vi "calc.vi"() -> ()   [LabVIEW 2011]
uses:
  global_vars.vi
  <vilib>/Utility/file.llb/Write To Spreadsheet File (I64).vi
panel:
  in  "b_calc_all":bool
  out "calculating":bool
  in  "calc \ndisplacement":bool
  in  "file path (dialog if empty)":path
  in  "dbl_gamma_correction":dbl=1.0
  in  "dbl_noise_threshold":dbl=20.0
  in  "update global variables":bool
  in  "safety margin":i32=5
  out "u8_ar_noise_mask":u8[][](array[numeric])
  in  "Tab Control":T1(tab)
  out "img_dist_input":T2(plugin-control)
  out "img_orig_input":T2(plugin-control)
  in  "i32_sel_input_image":i32
  in  "select row input":i32(slide) scale=-1.1..1049.0
  out "input_line_plot":dbl[][](graph)
  out "noise_mask_line_plot":u8[](graph)
  in  "select row noise map":i32(slide) scale=-1.1..1049.0
  out "last px":i32
  out "first px":i32
  out "img_noise_mask":T2(plugin-control)
  out "i32_First/last px":i32[][](graph)
  out "lineplot phasemap":dbl[][](graph)
  in  "select row phasemap":i32(slide) scale=0.0..1049.0
  out "img_dist_phaseMap":T2(plugin-control)
  out "img_orig_masked_with_dist":T2(plugin-control)
  out "img_dist_unwrap":T2(plugin-control)
  out "img_orig_unwrap":T2(plugin-control)
  in  "select row unwrapped":i32(slide) scale=-1.1..1049.0
  out "lineplot unwrapped":dbl[][](graph)
  out "graph_displacement":i32[][](graph)
  in  "select row displacement":i32(slide) scale=-1.1..1049.0
  out "lineplot displacement":i32[](graph)
  in  "save data":bool
  out "i32_ar_displacement":i32[][](array[numeric])
  in  "calc \nunwrapped\nphase map":bool
  out "Y Resolution":i32
  out "X Resolution":i32
  in  "update_cor":bool
  out "path_dist_files":path[](array[path])=[path "X:/Cloud Drives/Dropbox/Europhotonics/FringeMan/Image Storage/02_07/x-direction/dist/12_56_10-5.00fringes_0of4__capt_.png", path "X:/Cloud Drives/Dropbox/Europhotonics/FringeMan/Image Storage/02_07/x-direction/dist/12_56_10-5.00fringes_1of4__capt_.png", path "X:/Cloud Drives/Dropbox/Europhotonics/FringeMan/Image Storage/02_07/x-direction/dist/12_56_10-5.00fringes_2of4__capt_.png", path "X:/Cloud Drives/Dropbox/Europhotonics/FringeMan/Image Storage/02_07/x-direction/dist/12_56_10-5.00fringes_3of4__capt_.png"]
  out "path_orig_files":path[](array[path])=[path "X:/Cloud Drives/Dropbox/Europhotonics/FringeMan/Image Storage/02_07/x-direction/orig/12_56_10-5.00fringes_0of4__original_.png", path "X:/Cloud Drives/Dropbox/Europhotonics/FringeMan/Image Storage/02_07/x-direction/orig/12_56_10-5.00fringes_1of4__original_.png", path "X:/Cloud Drives/Dropbox/Europhotonics/FringeMan/Image Storage/02_07/x-direction/orig/12_56_10-5.00fringes_2of4__original_.png", path "X:/Cloud Drives/Dropbox/Europhotonics/FringeMan/Image Storage/02_07/x-direction/orig/12_56_10-5.00fringes_3of4__original_.png"]
  in  "dbl_ar_crop_correction":dbl[](array[numeric])=[0.0, 0.0, 0.0, 0.0] caption="crop_correction"
  in  "u8_y_center_cor":i16
  in  "u8_x_center_cor":i16=-20
  in  "radius correction":i16=-30
  out "u8_ar_orig_phasemap":dbl[][](array[numeric])
  out "dbl_pxar_orig_unwrap":dbl[][](array[numeric])
  out "dbl_pxar_dist_unwrap":dbl[][](array[numeric])
  out "u8_pxar_orig":dbl[][][](array[numeric])
  in  "read orig":bool
  in  "read dist":bool
  out "u8_ar_dist_phasemap":dbl[][](array[numeric])
  in  "calculate \nphase map":bool
  out "u8_pxar_dist":dbl[][][](array[numeric])
  in  "Stop Button":bool
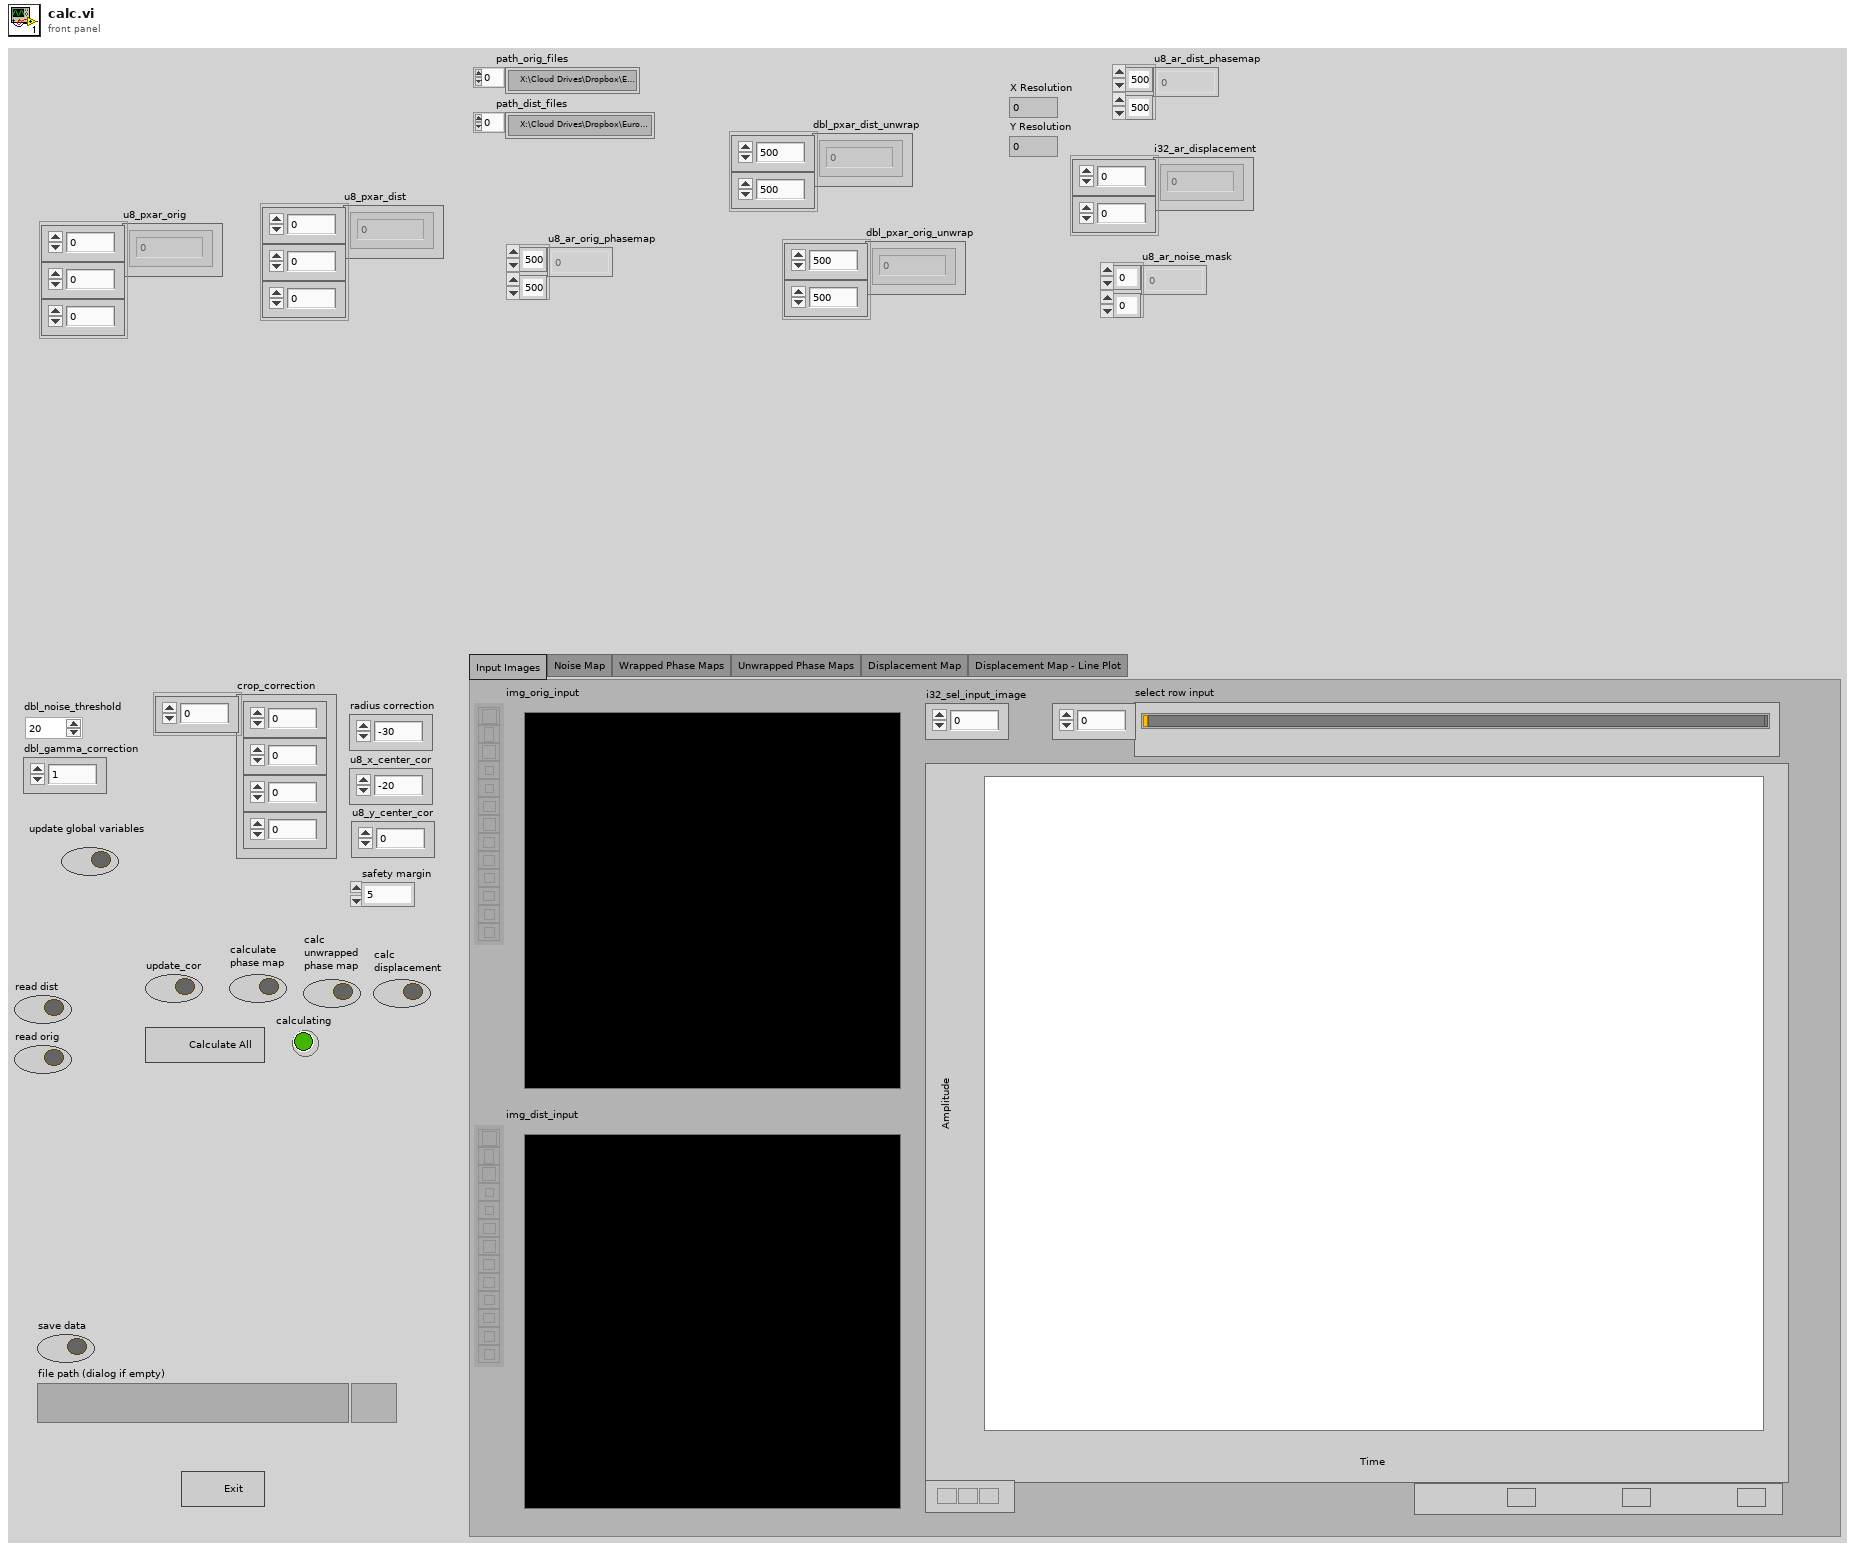
[diagram p1: front panel]
types:
  T1 = enum32{"Input Images", "Noise Map", "Wrapped Phase Maps", "Unwrapped Phase Maps", "Displacement Map", "Displacement Map - Line Plot"}
  T2 = typedef "IMAQ Image.ctl" = refnum<image>
  T3 = cluster{"radius correction":i16, "u8_x_center_cor":i16, "u8_y_center_cor":i16}
  T4 = typedef "Image Type" = u32
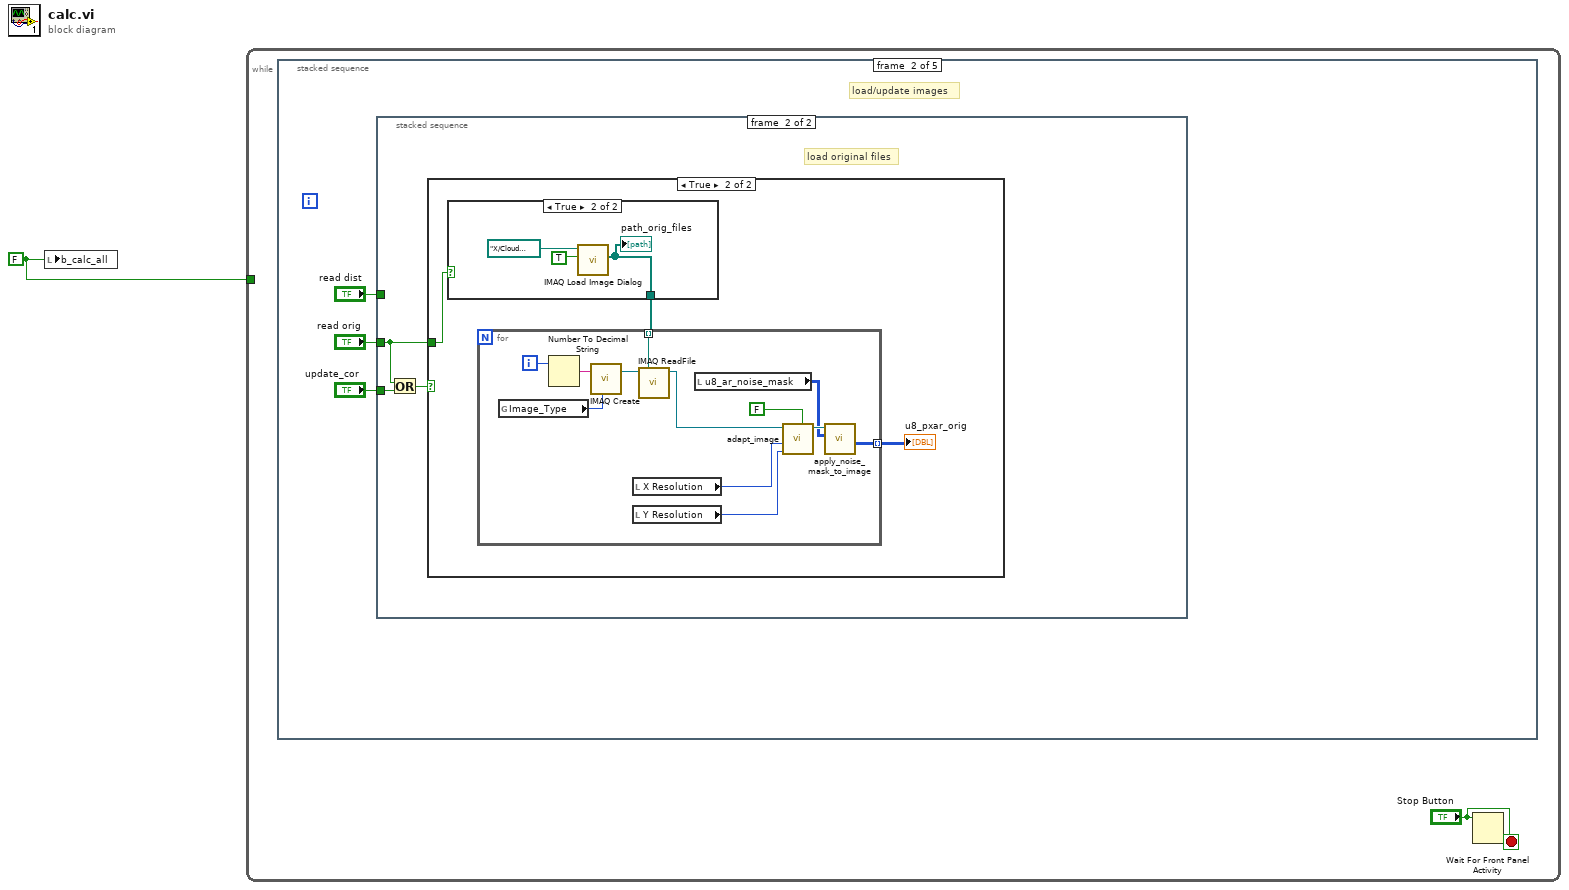
[diagram p0: block diagram]
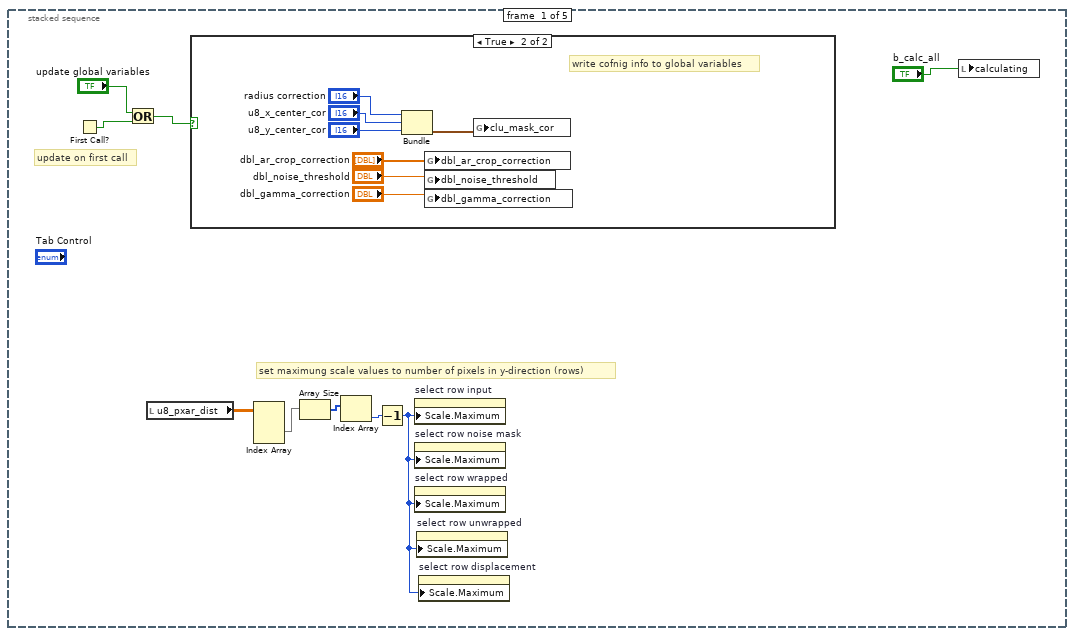
[diagram p2: hidden frame]
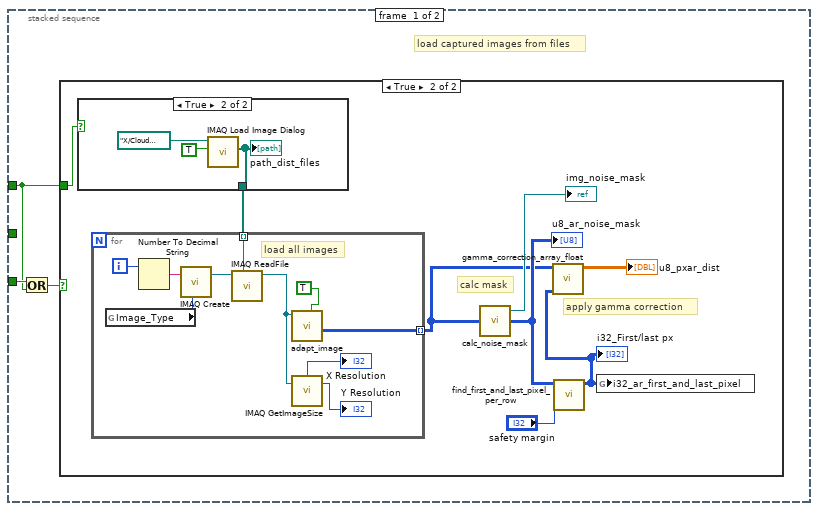
[diagram p4: hidden frame]
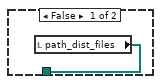
[diagram p6: hidden frame]
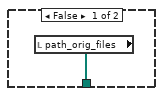
[diagram p8: hidden frame]
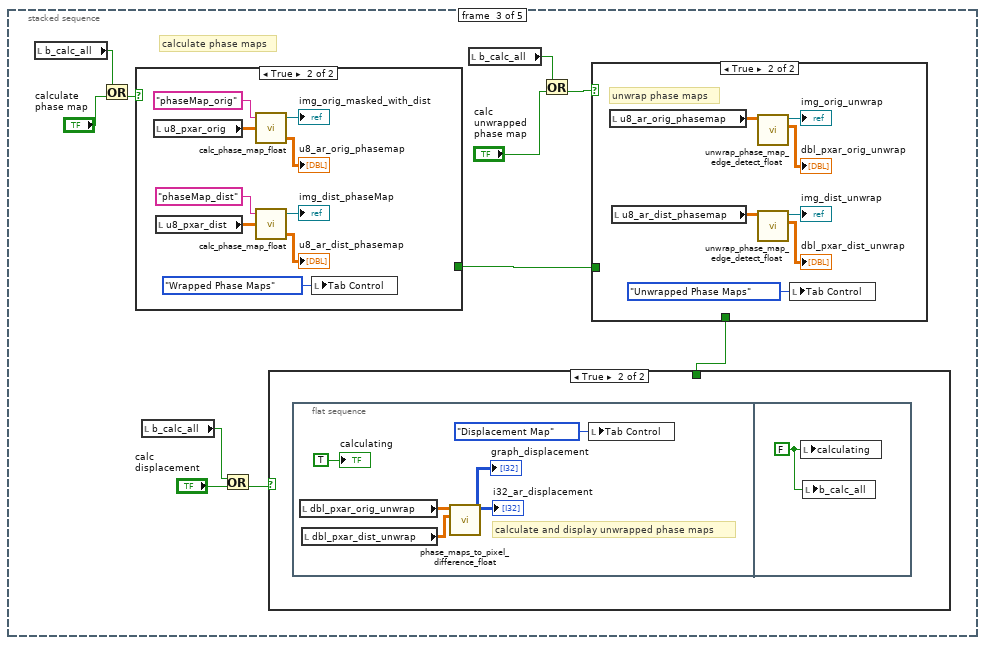
[diagram p9: hidden frame]
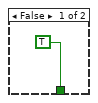
[diagram p11: hidden frame]
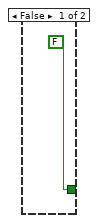
[diagram p12: hidden frame]
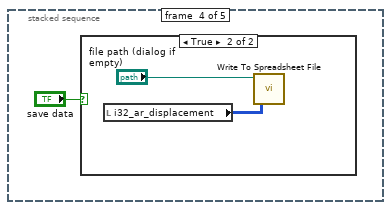
[diagram p13: hidden frame]
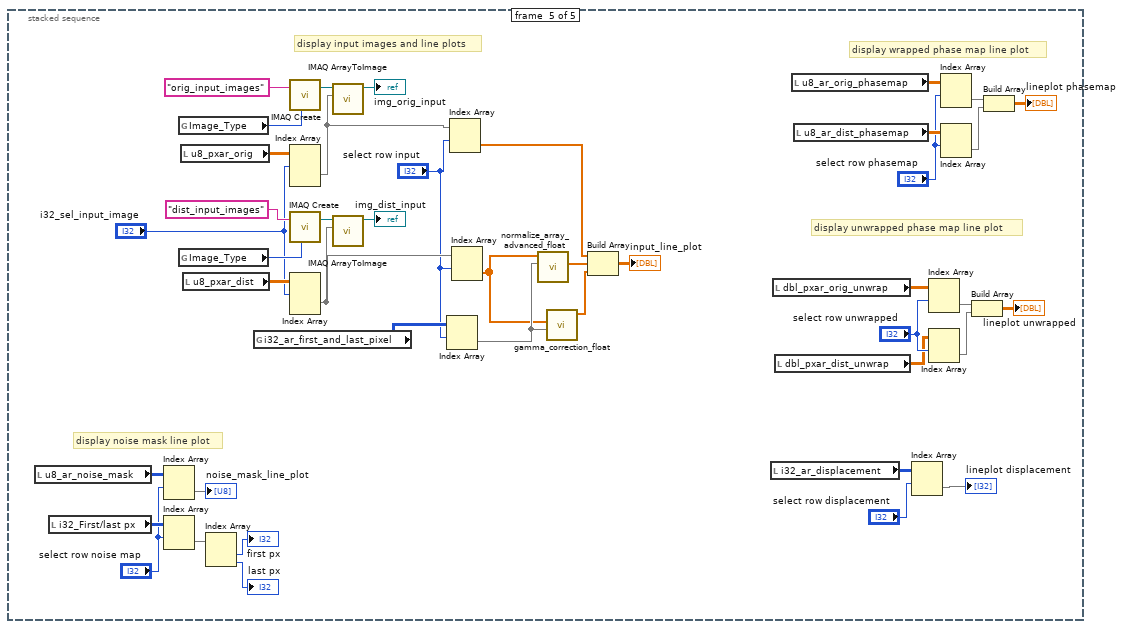
[diagram p15: hidden frame]
diagram:
  w1 = FALSE ("b_calculate all")
  n1 = local write "b_calc_all"(w1) -> ()
  n2 = while {
    tunnel: w1 -> [_]
    stop <- "Stop Button" stop-if-true
    n3 = stacked-sequence {
      frame #0 {
        # "set maximung scale values to number of pixels in y-direction (rows)"
        # "update on first call"
        n4 = First Call?() -> (First Call?: T/F=w9:bool)
        n5 = Or(x="update global variables", y=w9) -> (x .or. y?=w10:bool)
        n6 = local read "u8_pxar_dist"() -> (w7:dbl[][][])
        n7 = case shown="True" w10 {
          frame False {
          }
          frame True {
            # "write cofnig info to global variables"
            n8 = Bundle("radius correction"="radius correction", "u8_x_center_cor"="u8_x_center_cor", "u8_y_center_cor"="u8_y_center_cor") -> (w18:T3)  [unwired: 1 in]
            n9 = global write "global_vars.vi" "dbl_ar_crop_correction"("dbl_ar_crop_correction") -> ()
            n10 = global write "global_vars.vi" "dbl_noise_threshold"("dbl_noise_threshold") -> ()
            n11 = global write "global_vars.vi" "dbl_gamma_correction"("dbl_gamma_correction") -> ()
            n12 = global write "global_vars.vi" "clu_mask_cor"(w18) -> ()
          }
        }
        n13 = Index Array(array=w7) -> (element=w8:dbl[][])  [unwired: 3 in]
        n14 = Array Size(array=w8) -> (size(s)=w6:i32[])
        n15 = Index Array(array=w6) -> (element=w5:i32)  [unwired: 1 in]
        n16 = Decrement(x=w5) -> (x-1=w4:i32)
        n17 = property on="select row input" class="Slide (strict)"("Scale.Maximum"=w4) -> ()  [unwired: 2 in, 2 out]
        n18 = property on="select row noise mask" class="Slide (strict)"("Scale.Maximum"=w4) -> ()  [unwired: 2 in, 2 out]
        n19 = property on="select row wrapped" class="Slide (strict)"("Scale.Maximum"=w4) -> ()  [unwired: 2 in, 2 out]
        n20 = property on="select row unwrapped" class="Slide (strict)"("Scale.Maximum"=w4) -> ()  [unwired: 2 in, 2 out]
        n21 = property on="select row displacement" class="Slide (strict)"("Scale.Maximum"=w4) -> ()  [unwired: 2 in, 2 out]
        n22 = local write "calculating"("b_calc_all") -> ()
      }
      frame #1 {
        # "load/update images"
        n23 = stacked-sequence {
          tunnel: "update_cor" -> [w24 w48]
          tunnel: "read dist" -> [w22 _]
          tunnel: "read orig" -> [_ w47]
          frame #0 {
            # "load captured images from files"
            n24 = Or(x=w24, y=w22) -> (x .or. y?=w23:bool)
            n25 = case shown="True" w23 {
              tunnel: w22 -> [_ w31]
              frame False {
              }
              frame True {
                # "apply gamma correction"
                # "calc mask"
                n26 = case shown="True" w31 {
                  tunnel: [w33 w36] -> w32
                  frame False {
                    n27 = local read "path_dist_files"() -> (w33:path[])
                  }
                  frame True {
                    n28 = call "IMAQ Load Image Dialog"("Multiple Files? (No)"=TRUE, "Start Path"=path "X:/Cloud Drives/Dropbox/Europhotonics/FringeMan/Image Storage") -> ("Paths"=w36:path[])  [unwired: 7 in, 2 out]
                    "path_dist_files" <- w36
                  }
                }
                n29 = for {
                  tunnel: w32 -> [w42] mode=indexing
                  tunnel: [w38] -> w27 mode=indexing
                  i -> [w46]
                  # "load all images"
                  n30 = global read "global_vars.vi" "Image_Type"() -> (w43:T4)
                  n31 = Number To Decimal String(number=w46) -> (decimal integer string=w45:string)  [unwired: 1 in]
                  n32 = call "IMAQ Create"("Image Name"=w45, "Image Type"=w43) -> ("New Image"=w44:T2)  [unwired: 2 in, 2 out]
                  n33 = call "IMAQ ReadFile"("File Path"=w42, "Image"=w44) -> ("Image Out"=w39:T2)  [unwired: 5 in, 4 out]
                  n34 = call "adapt_image.vi"("captured image?"=TRUE, "orig_imageIn"=w39) -> ("adapted image px array"=w38:u8[][])  [unwired: 7 in, 2 out]
                  n35 = call "IMAQ GetImageSize"("Image"=w39) -> ("Y Resolution"=→"Y Resolution":i32, "X Resolution"=→"X Resolution":i32)  [unwired: 3 in, 1 out]
                }
                n36 = call "calc_noise_mask.vi"("u8_ar_image_pixel_array"=w27) -> ("u8_ar_noise_mask"=w28:u8[][], "img_noise mask"=→"img_noise_mask":T2)  [unwired: 3 in]
                "u8_ar_noise_mask" <- w28
                n37 = call "find_first_and_last_pixel_per_row.vi"("safety margin"="safety margin", "u8_ar_mask"=w28) -> ("i32_ar_first_and_last_pixel"=w25:i32[][])  [unwired: 9 in]
                "i32_First/last px" <- w25
                n38 = call "gamma_correction_array_float.vi"("i32_ar_first_and_last_pixel"=w25, "adapted image px array"=w27) -> ("i16_normalized unwrapped array"=→"u8_pxar_dist":dbl[][][])  [unwired: 9 in]
                n39 = global write "global_vars.vi" "i32_ar_first_and_last_pixel"(w25) -> ()
              }
            }
          }
          frame #1 {
            # "load original files"
            n40 = Or(x=w47, y=w48) -> (x .or. y?=w49:bool)
            n41 = case shown="True" w49 {
              tunnel: w47 -> [_ w51]
              frame False {
              }
              frame True {
                n42 = case shown="True" w51 {
                  tunnel: [w53 w55] -> w52
                  frame False {
                    n43 = local read "path_orig_files"() -> (w53:path[])
                  }
                  frame True {
                    n44 = call "IMAQ Load Image Dialog"("Multiple Files? (No)"=TRUE, "Start Path"=path "X:/Cloud Drives/Dropbox/Europhotonics/FringeMan/Image Storage") -> ("Paths"=w55:path[])  [unwired: 7 in, 2 out]
                    "path_orig_files" <- w55
                  }
                }
                n45 = for {
                  tunnel: w52 -> [w68] mode=indexing
                  tunnel: [w58] -> w50 mode=indexing
                  i -> [w64]
                  n46 = global read "global_vars.vi" "Image_Type"() -> (w65:T4)
                  n47 = Number To Decimal String(number=w64) -> (decimal integer string=w67:string)  [unwired: 1 in]
                  n48 = call "IMAQ Create"("Image Name"=w67, "Image Type"=w65) -> ("New Image"=w66:T2)  [unwired: 2 in, 2 out]
                  n49 = local read "X Resolution"() -> (w62:i32)
                  n50 = local read "Y Resolution"() -> (w61:i32)
                  n51 = call "IMAQ ReadFile"("File Path"=w68, "Image"=w66) -> ("Image Out"=w63:T2)  [unwired: 5 in, 4 out]
                  n52 = local read "u8_ar_noise_mask"() -> (w57:u8[][])
                  n53 = call "adapt_image.vi"("captured image?"=FALSE, "captImage_Y_Resolution"=w61, "captImage_X_Resolution"=w62, "orig_imageIn"=w63) -> ("adapted image"=w59:T2)  [unwired: 5 in, 2 out]
                  n54 = call "apply_noise_mask_to_image.vi"("u8_ar_noise_mask in"=w57, "Refnum in"=w59) -> ("Image Pixels (U8)"=w58:u8[][])  [unwired: 7 in, 2 out]
                }
                "u8_pxar_orig" <- w50
              }
            }
          }
        }
      }
      frame #2 {
        # "calculate phase maps"
        n55 = local read "b_calc_all"() -> (w71:bool)
        n56 = Or(x=w71, y="calculate \nphase map") -> (x .or. y?=w74:bool)
        n57 = case shown="True" w74 {
          tunnel: [FALSE _] -> w77
          frame False {
          }
          frame True {
            n58 = local read "u8_pxar_orig"() -> (w98:dbl[][][])
            n59 = local read "u8_pxar_dist"() -> (w102:dbl[][][])
            n60 = call "calc_phase_map_float.vi"("u8_ar_image_pixel_array"=w98, "image name"="phaseMap_orig" ("String")) -> ("raw phase map array"=→"u8_ar_orig_phasemap":dbl[][], "phase map"=→"img_orig_masked_with_dist":T2)  [unwired: 2 in]
            n61 = call "calc_phase_map_float.vi"("u8_ar_image_pixel_array"=w102, "image name"="phaseMap_dist" ("String")) -> ("raw phase map array"=→"u8_ar_dist_phasemap":dbl[][], "phase map"=→"img_dist_phaseMap":T2)  [unwired: 2 in]
            n62 = local write "Tab Control"(T1."Wrapped Phase Maps" ("Tab Control")) -> ()
          }
        }
        n63 = local read "b_calc_all"() -> (w69:bool)
        n64 = Or(x=w69, y="calc \ndisplacement") -> (x .or. y?=w72:bool)
        n65 = local read "b_calc_all"() -> (w70:bool)
        n66 = Or(x=w70, y="calc \nunwrapped\nphase map") -> (x .or. y?=w73:bool)
        n67 = case shown="True" w73 {
          tunnel: w77 -> [_ _]
          tunnel: [TRUE _] -> w75
          frame False {
          }
          frame True {
            # "unwrap phase maps"
            n68 = local read "u8_ar_orig_phasemap"() -> (w90:dbl[][])
            n69 = local read "u8_ar_dist_phasemap"() -> (w91:dbl[][])
            n70 = call "unwrap_phase_map_edge_detect_float.vi"("u8_ar_dist_phasemap"=w90) -> ("df_ar_unwrapped_px_ar"=→"dbl_pxar_orig_unwrap":dbl[][], "Refnum out"=→"img_orig_unwrap":T2)  [unwired: 9 in]
            n71 = call "unwrap_phase_map_edge_detect_float.vi"("u8_ar_dist_phasemap"=w91) -> ("df_ar_unwrapped_px_ar"=→"dbl_pxar_dist_unwrap":dbl[][], "Refnum out"=→"img_dist_unwrap":T2)  [unwired: 9 in]
            n72 = local write "Tab Control"(T1."Unwrapped Phase Maps" ("Tab Control")) -> ()
          }
        }
        n73 = case shown="True" w72 {
          tunnel: w75 -> [_ _]
          frame False {
          }
          frame True {
            n74 = flat-sequence {
              frame #0 {
                # "calculate and display unwrapped phase maps"
                n75 = local read "dbl_pxar_orig_unwrap"() -> (w82:dbl[][])
                n76 = local read "dbl_pxar_dist_unwrap"() -> (w83:dbl[][])
                n77 = call "phase_maps_to_pixel_difference_float.vi"("dist phase map"=w83, "oirg phase map"=w82) -> ("displacement map"=→"i32_ar_displacement" →"graph_displacement":i32[][])  [unwired: 9 in]
                n78 = local write "Tab Control"(T1."Displacement Map" ("Tab Control")) -> ()
                "calculating" <- TRUE
              }
              frame #1 {
                w85 = FALSE
                n79 = local write "calculating"(w85) -> ()
                n80 = local write "b_calc_all"(w85) -> ()
              }
            }
          }
        }
      }
      frame #3 {
        n81 = case shown="True" "save data" {
          frame False {
          }
          frame True {
            n82 = local read "i32_ar_displacement"() -> (w106:i32[][])
            n83 = call-poly <vilib>:"Write To Spreadsheet File.vi"("2D data"=w106, "file path (dialog if empty)"="file path (dialog if empty)") -> ()  [unwired: 6 in, 1 out]
          }
        }
      }
      frame #4 {
        # "display unwrapped phase map line plot"
        # "display noise mask line plot"
        # "display wrapped phase map line plot"
        # "display input images and line plots"
        n84 = local read "u8_ar_noise_mask"() -> (w143:u8[][])
        n85 = local read "i32_First/last px"() -> (w138:i32[][])
        n86 = Index Array(array=w143, index (row)="select row noise map") -> (element=→"noise_mask_line_plot":u8[])  [unwired: 1 in]
        n87 = Index Array(array=w138, index (row)="select row noise map") -> (element=w139:i32[])  [unwired: 1 in]
        n88 = global read "global_vars.vi" "Image_Type"() -> (w133:T4)
        n89 = global read "global_vars.vi" "Image_Type"() -> (w130:T4)
        n90 = local read "u8_pxar_orig"() -> (w134:dbl[][][])
        n91 = local read "u8_pxar_dist"() -> (w135:dbl[][][])
        n92 = Index Array(array=w139) -> (element #1=→"first px":i32, element #2=→"last px":i32)  [unwired: 2 in]
        n93 = global read "global_vars.vi" "i32_ar_first_and_last_pixel"() -> (w124:i32[][])
        n94 = call "IMAQ Create"("Image Name"="orig_input_images", "Image Type"=w133) -> ("New Image"=w128:T2)  [unwired: 2 in, 2 out]
        n95 = Index Array(array=w134, index (dim 0)="i32_sel_input_image") -> (element=w125:dbl[][])  [unwired: 2 in]
        n96 = call "IMAQ Create"("Image Name"="dist_input_images", "Image Type"=w130) -> ("New Image"=w129:T2)  [unwired: 2 in, 2 out]
        n97 = Index Array(array=w135, index (dim 0)="i32_sel_input_image") -> (element=w136:dbl[][])  [unwired: 2 in]
        n98 = call "IMAQ ArrayToImage"("Image Pixels (U8)"=w125, "Image"=w128) -> ("Image Out"=→"img_orig_input":T2)  [unwired: 8 in, 1 out]
        n99 = call "IMAQ ArrayToImage"("Image Pixels (U8)"=w136, "Image"=w129) -> ("Image Out"=→"img_dist_input":T2)  [unwired: 8 in, 1 out]
        n100 = Index Array(array=w124, index (row)="select row input") -> (element=w120:i32[])  [unwired: 1 in]
        n101 = Index Array(array=w125, index (row)="select row input") -> (element=w118:dbl[])  [unwired: 1 in]
        n102 = Index Array(array=w136, index (row)="select row input") -> (element=w116:dbl[])  [unwired: 1 in]
        n103 = call "normalize_array_advanced_float.vi"("i32_ar_first_and_last_pixel"=w120, "unwrapped array"=w116) -> ("i16_normalized unwrapped array"=w117:dbl[])  [unwired: 5 in, 4 out]
        n104 = call "gamma_correction_float.vi"("i32_ar_first_and_last_pixel"=w120, "u8_pxar_dist"=w116) -> ("i16_normalized unwrapped array"=w119:dbl[])  [unwired: 9 in]
        n105 = Build Array(w118, w117, w119) -> (→"input_line_plot":dbl[][])
        n106 = local read "i32_ar_displacement"() -> (w109:i32[][])
        n107 = local read "dbl_pxar_orig_unwrap"() -> (w111:dbl[][])
        n108 = local read "dbl_pxar_dist_unwrap"() -> (w110:dbl[][])
        n109 = local read "u8_ar_orig_phasemap"() -> (w149:dbl[][])
        n110 = local read "u8_ar_dist_phasemap"() -> (w148:dbl[][])
        n111 = Index Array(array=w109, index (row)="select row displacement") -> (element=→"lineplot displacement":i32[])  [unwired: 1 in]
        n112 = Index Array(array=w111, index (row)="select row unwrapped") -> (element=w115:dbl[])  [unwired: 1 in]
        n113 = Index Array(array=w110, index (row)="select row unwrapped") -> (element=w114:dbl[])  [unwired: 1 in]
        n114 = Index Array(array=w149, index (row)="select row phasemap") -> (element=w146:dbl[])  [unwired: 1 in]
        n115 = Index Array(array=w148, index (row)="select row phasemap") -> (element=w145:dbl[])  [unwired: 1 in]
        n116 = Build Array(w115, w114) -> (→"lineplot unwrapped":dbl[][])
        n117 = Build Array(w146, w145) -> (→"lineplot phasemap":dbl[][])
      }
    }
    n118 = Wait For Front Panel Activity(3:"Stop Button") -> ()  [unwired: 2 in, 1 out]
  }
